vi "Read Ignore Case.vi"(8 "error in (no error)":errorcluster, 11 "String Compare in":refnum<class "String Compare.lvclass">) -> (0 "error out":errorcluster, 2 "ignore case? (F)":bool, 3 "String Compare out":refnum<class "String Compare.lvclass">)   [LabVIEW 2015, in "String Compare.lvclass"]
uses:
  String Compare.lvclass
  String Compare.lvclass/String Compare.ctl
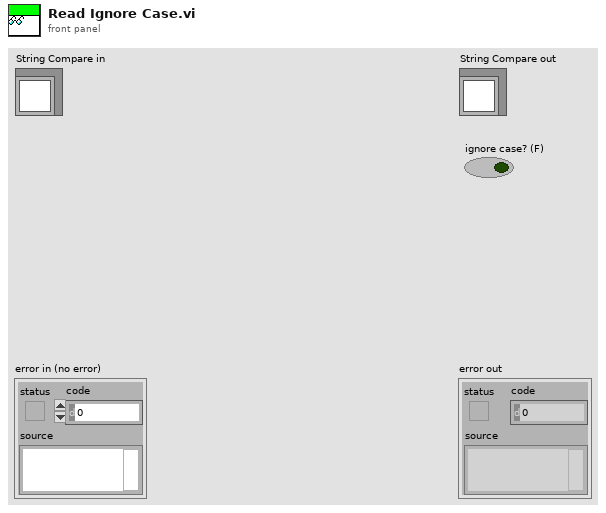
[diagram p1: front panel]
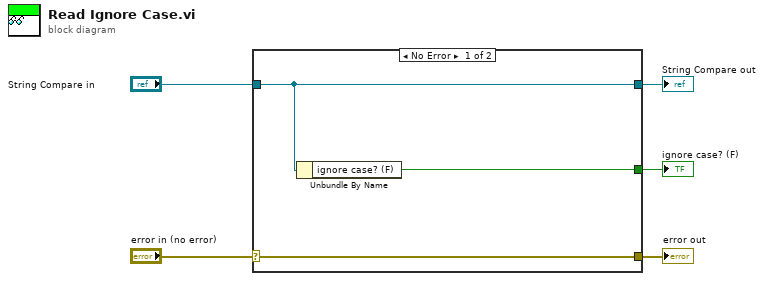
[diagram p0: block diagram]
diagram:
  n1 = case shown="No Error" "error in (no error)" {
    selector: "error in (no error)" -> [w8 w9]
    tunnel: [w8 w9] -> w4
    tunnel: [w7 w10] -> w2
    tunnel: "String Compare in" -> [w7 w10]
    tunnel: [w6 _] -> w1
    frame No Error {
      n2 = Unbundle By Name(w7) -> ("ignore case? (F)"=w6:bool)
    }
    frame Error {
    }
  }
  "error out" <- w4
  "String Compare out" <- w2
  "ignore case? (F)" <- w1
